vi "Generate IMU Calibration Array.vi"(1 "Read Bearing (0-360 degrees)":dbl[](array[numeric])=[30.0, 150.0, 180.0, 300.0, 390.0], 2 "Actual Bearing (0-360 degrees)":dbl[](array[numeric])=[0.0, 90.0, 180.0, 270.0, 360.0]) -> (0 "Bearing modification":dbl[](graph)=[-30.0, -29.0, -28.0, -27.0, -26.0, -25.0, -24.0, -23.0, -22.0, -21.0, -20.0, -19.0, -18.0, -17.0, -16.0, -15.0, -14.0, -13.0, -12.0, -11.0, -10.0, -9.0, -8.0, -7.0, -6.0, -5.0, -4.0, -3.0, -2.0, -1.0, 0.0, 0.75, 1.5, 2.25, 3.0, 3.75, 4.5, 5.25, 6.0, 6.75, 7.5, 8.25, 9.0, 9.75, 10.5, 11.25, 12.0, 12.75, 13.5, 14.25, 15.0, 15.749999999999998, 16.5, 17.25, 18.0, 18.75, 19.5, 20.25, 21.0, 21.75, 22.5, 23.250000000000004, 24.0, 24.750000000000004, 25.5, 26.25, 27.0, 27.75, 28.5, 29.25, 30.0, 30.75, 31.499999999999996, 32.25, 33.0, 33.75, 34.5, 35.25, 36.0, 36.75, 37.5, 38.25, 39.0, 39.75, 40.5, 41.25, 42.0, 42.75, 43.5, 44.25, 45.0, 45.75, 46.50000000000001, 47.25, 48.0, 48.75, 49.50000000000001, 50.25, 51.0, 51.74999999999999, 52.5, 53.25, 54.0, 54.74999999999999, 55.5, 56.25, 57.0, 57.75000000000001, 58.5, 59.25, 60.0, 60.75000000000001, 61.5, 62.25, 62.99999999999999, 63.75, 64.5, 65.25, 66.0, 66.75, 67.5, 68.25, 69.0, 69.75, 70.5, 71.25, 72.0, 72.75, 73.5, 74.25, 75.0, 75.75, 76.5, 77.25, 78.0, 78.75, 79.5, 80.25, 81.0, 81.75, 82.5, 83.25, 84.0, 84.75, 85.5, 86.25, 87.0, 87.75, 88.5, 89.25, 90.0, 93.0, 96.0, 99.0, 102.0, 105.0, 108.0, 111.0, 114.0, 117.0, 120.0, 123.0, 126.0, 129.0, 132.0, 135.0, 138.0, 141.0, 144.0, 147.0, 150.0, 153.0, 156.0, 159.0, 162.0, 165.0, 168.0, 171.0, 174.0, 177.0, 180.0, -179.25, -178.5, -177.75, -177.0, -176.25, -175.5, -174.75, -174.0, -173.25, -172.5, -171.75, -171.0, -170.25, -169.5, -168.75, -168.0, -167.25, -166.5, -165.75, -165.0, -164.25, -163.5, -162.75, -162.0, -161.25, -160.5, -159.75, -159.0, -158.25, -157.5, -156.75, -156.0, -155.25, -154.5, -153.75, -153.0, -152.25, -151.5, -150.75, -150.0, -149.25, -148.5, -147.75, -147.0, -146.25, -145.5, -144.75, -144.0, -143.25, -142.5, -141.75, -141.0, -140.25, -139.5, -138.75, -138.0, -137.25, -136.5, -135.75, -135.0, -134.25, -133.5, -132.75, -132.0, -131.25, -130.5, -129.75, -129.0, -128.25, -127.5, -126.75, -126.0, -125.25, -124.5, -123.75, -123.0, -122.25, -121.5, -120.75, -120.0, -119.25, -118.5, -117.75, -117.0, -116.25, -115.5, -114.75, -114.0, -113.25, -112.5, -111.75, -111.0, -110.25, -109.5, -108.75, -108.0, -107.25, -106.5, -105.75, -105.0, -104.25, -103.5, -102.75, -102.0, -101.25, -100.5, -99.75, -99.0, -98.25, -97.5, -96.75, -96.0, -95.25, -94.5, -93.75, -93.0, -92.25, -91.5, -90.75, -90.0, -89.0, -88.0, -87.0, -86.0, -85.0, -84.0, -83.0, -82.0, -81.0, -80.0, -79.0, -78.0, -77.0, -76.0, -75.0, -74.0, -73.0, -72.0, -71.0, -70.0, -69.0, -68.0, -67.0, -66.0, -65.0, -64.0, -63.0, -62.0, -61.0, -60.0, -59.0, -58.0, -57.0, -56.0, -55.0, -54.0, -53.0, -52.0, -51.0, -50.0, -49.0, -48.0, -47.0, -46.0, -45.0, -44.0, -43.0, -42.0, -41.0, -40.0, -39.0, -38.0, -37.0, -36.0, -35.0, -34.0, -33.0, -32.0, -31.0])   [LabVIEW 2011]
uses:
  <vilib>/Analysis/coordinate.llb/Angle Units.ctl
  <vilib>/Analysis/coordinate.llb/Angle Range (Degree).ctl
  <vilib>/Analysis/coordinate.llb/Wrap Angle (array).vi
  <vilib>/Analysis/NI_AAL_Angle.lvlib
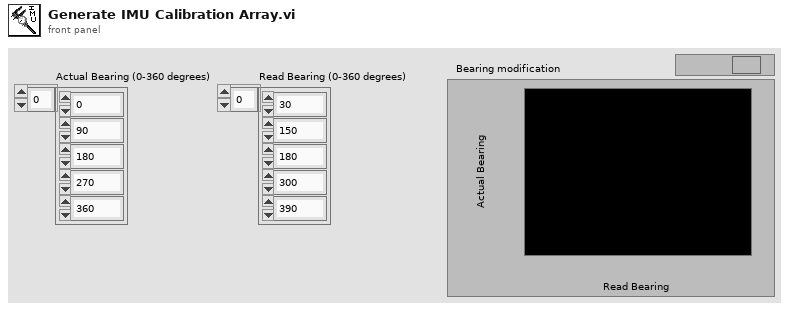
[diagram p1: front panel]
types:
  T1 = typedef "NI_AAL_Angle.lvlib/Angle Range (Degree).ctl" = u16
  T2 = typedef "NI_AAL_Angle.lvlib/Angle Units.ctl" = i32
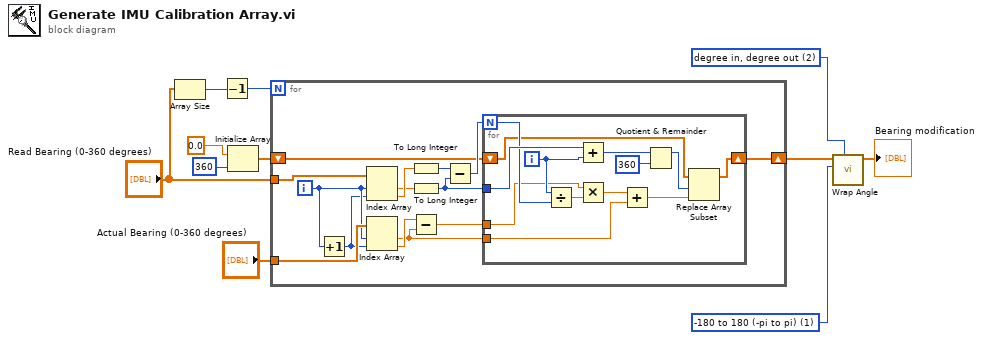
[diagram p0: block diagram]
diagram:
  w4 = T1 1 items=["none", "-180 to 180 (-pi to pi)", "0 to 360 (0 to 2pi)"] ("angle range")
  w3 = T2 2 items=["radian in, radian out", "radian in, degree out", "degree in, degree out", "degree in, radian out"] ("angle units")
  n1 = Array Size(array="Read Bearing (0-360 degrees)") -> (size(s)=w11:i32)
  n2 = Decrement(x=w11) -> (x-1=w6:i32)
  n3 = Initialize Array(0.0 ("element"), 360 ("dimension size")) -> (w5:dbl[])
  n4 = for {
    N: w6 -> [_]
    tunnel: "Read Bearing (0-360 degrees)" -> [w25]
    tunnel: "Actual Bearing (0-360 degrees)" -> [w24]
    shift-right: [w13] -> w2
    shift-left: w5 -> [w14]
    i -> [w23]
    n5 = Increment(x=w23) -> (x+1=w22:i32)
    n6 = Index Array(array=w25, index #1=w23, index #2=w22) -> (element #1=w20:dbl, element #2=w21:dbl)
    n7 = Index Array(array=w24, index #1=w23, index #2=w22) -> (element #1=w12:dbl, element #2=w16:dbl)
    n8 = To Long Integer(number=w21) -> (32bit integer=w19:i32)
    n9 = To Long Integer(number=w20) -> (32bit integer=w17:i32)
    n10 = Subtract(x=w16, y=w12) -> (x-y=w15:dbl)
    n11 = Subtract(x=w19, y=w17) -> (x-y=w18:i32)
    n12 = for {
      N: w18 -> [w36]
      tunnel: w17 -> [w38]
      tunnel: w15 -> [w34]
      shift-right: [w32] -> w13
      shift-left: w14 -> [w33]
      tunnel: w12 -> [w29]
      i -> [w37]
      n13 = Divide(x=w37, y=w36) -> (x/y=w35:dbl)
      n14 = Add(x=w38, y=w37) -> (x+y=w28:i32)
      n15 = Multiply(x=w34, y=w35) -> (x*y=w31:dbl)
      n16 = Add(x=w31, y=w29) -> (x+y=w30:dbl)
      n17 = Quotient & Remainder(x=w28, y=360) -> (x-y*floor(x/y)=w26:i32)  [unwired: 1 out]
      n18 = Replace Array Subset(array=w33, new element=w30, index=w26) -> (w32:dbl[])
    }
  }
  n19 = call-poly <vilib>:"Wrap Angle.vi"("angle units"=w3, "angle range"=w4, "Angle In"=w2) -> ("Angle Out"=→"Bearing modification":dbl[])  [unwired: 7 in, 1 out]
